vi "Actor Core.vi"(8 "error in":errorcluster, 11 "hydraharp_panel in":refnum<class "tt20panel.lvclass">) -> (0 "error out":errorcluster, 3 "Actor out":refnum<class "Actor.lvclass">)   [LabVIEW 2015, in "tt20panel.lvclass"]
doc: "(<B>Filename</B>: Actor Framework.lvlib:Actor.lvclass:Actor Core.vi)\n\nReceives messages to the actor, reacts to them, and initiates any error handling that may shut the actor down.\n\nDescendant classes may override this VI to append parallel tasks for the actor to complete while it handles messages. Overrides use the Call Parent Method node."
uses:
  tt20panel.lvclass
  <vilib>/ActorFramework/Actor/Actor.lvclass
  tt20_tasks_tdef.ctl
  tt20_settings_tdef.ctl
  tt20_ch_settings_tdef.ctl
  tt20_acq_mode_tdef.ctl
  UI/panel_class/panel.lvclass/panel.ctl
  <vilib>/ActorFramework/Actor/Actor.lvclass/Actor.ctl
  <vilib>/ActorFramework/Message Enqueuer/Message Enqueuer.lvclass/Message Enqueuer.ctl
  tt20panel.lvclass/tt20panel.ctl
  tt20_class/tt20_hardware_info_tdef.ctl
  tt20panel Messages/tt20panel_connect Msg/tt20panel_connect Msg.lvclass/tt20panel_connect Msg.ctl
  tt20panel Messages/tt20panel_DO_apply_settings Msg/tt20panel_DO_apply_settings Msg.lvclass/tt20panel_DO_apply_settings Msg.ctl
  tt20panel Messages/tt20panel_DO_chart_counts Msg/tt20panel_DO_chart_counts Msg.lvclass/tt20panel_DO_chart_counts Msg.ctl
  tt20_class/tt20_histo_settings_tdef.ctl
  tt20panel Messages/tt20panel_lifetime Msg/tt20panel_lifetime Msg.lvclass/tt20panel_lifetime Msg.ctl
  tt20panel Messages/tt20panel_correlate Msg/tt20panel_correlate Msg.lvclass/tt20panel_correlate Msg.ctl
  tt20_stream_settings_tdef.ctl
  tt20panel Messages/tt20panel_DO_stream_data Msg/tt20panel_DO_stream_data Msg.lvclass/tt20panel_DO_stream_data Msg.ctl
  <vilib>/ActorFramework/Message Enqueuer/Init from Existing Queue.vi
  <vilib>/ActorFramework/Message Enqueuer/Enqueue.vi
  <vilib>/ActorFramework/Message Priority Queue/Priority Enqueue.vi
  <vilib>/ActorFramework/Message Enqueuer/Message Enqueuer.lvclass
  tt20panel Messages/tt20panel_DO_disconnect Msg/tt20panel_DO_disconnect Msg.lvclass
  tt20panel Messages/tt20panel_connect Msg/tt20panel_connect Msg.lvclass
  tt20panel Messages/tt20panel_DO_apply_settings Msg/tt20panel_DO_apply_settings Msg.lvclass
  tt20panel Messages/tt20panel_DO_chart_counts Msg/tt20panel_DO_chart_counts Msg.lvclass
  tt20panel Messages/tt20panel_lifetime Msg/tt20panel_lifetime Msg.lvclass
  tt20panel Messages/tt20panel_correlate Msg/tt20panel_correlate Msg.lvclass
  tt20panel Messages/tt20panel_DO_stream_data Msg/tt20panel_DO_stream_data Msg.lvclass
  UI/panel_class/panel.lvclass
panel:
  in  "save_settings":bool
  in  "connect":bool
  out "Status":string
  out "error out 2":errorcluster
  in  "stop_task":bool
  in  "do_task":bool
  in  "Task":T1
  in  "tt20_tab":enum32{"Basic Settings", "File Stream"}(tab)
  in  "Number of Bins":i64
  in  "Bin Width (ps)":i64
  in  "Mode":T2
  out "Ch5":dbl
  out "Ch6":dbl
  out "Ch7":dbl
  in  "tt20_settings":T3=[{"enable"=TRUE, "trigger_level"=0.0, "deadtime_ns"=6, "delay_ps"=0}, {"enable"=TRUE, "trigger_level"=1.5, "deadtime_ns"=6, "delay_ps"=0}, {"enable"=TRUE, "trigger_level"=1.5, "deadtime_ns"=6, "delay_ps"=0}, {"enable"=FALSE, "trigger_level"=1.5, "deadtime_ns"=6, "delay_ps"=0}, {"enable"=FALSE, "trigger_level"=1.5, "deadtime_ns"=6, "delay_ps"=0}, {"enable"=FALSE, "trigger_level"=1.5, "deadtime_ns"=6, "delay_ps"=0}, {"enable"=FALSE, "trigger_level"=1.5, "deadtime_ns"=6, "delay_ps"=0}, {"enable"=FALSE, "trigger_level"=1.5, "deadtime_ns"=6, "delay_ps"=0}] {"trigger_level" min=0.0 max=5.0}
  out "Ch0":dbl
  out "Ch1":dbl
  out "Ch2":dbl
  out "Ch3":dbl
  out "Ch4":dbl
  in  "Reference Channel":u8 max=7 step=1
  in  "Stream Path":path
  in  "acq_time (s)":u32=1000
  in  "Stream Notes":string
  # "Time Tagger 20"
  # "Counts/s"
  # "Enable"
  # "Trig Lvl (V)"
  # "Dedtime (ns)"
  # "Delay (ps)"
  # "Stream Settings"
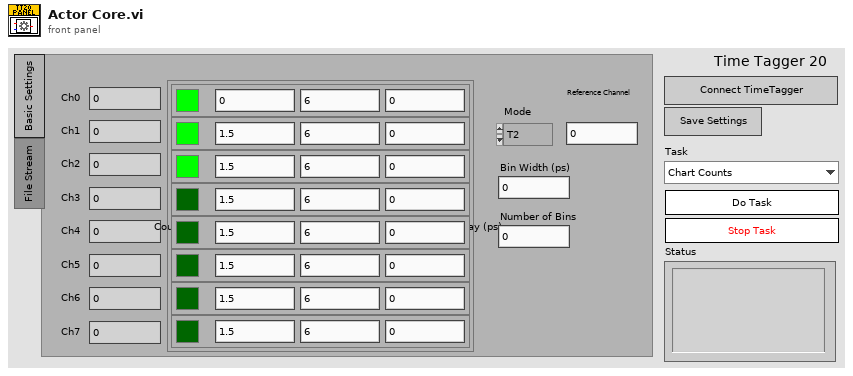
[diagram p1: front panel]
types:
  T1 = typedef "tt20_tasks_tdef.ctl" = enum16{"Chart Counts", "Stream to File", "Lifetime", "Correlate"}
  T2 = typedef "tt20_acq_mode_tdef.ctl" = enum16{"T2", "T3"}
  T3 = typedef "tt20_settings_tdef.ctl" = T4[]
  T4 = typedef "tt20_ch_settings_tdef.ctl" = cluster{"enable":bool, "trigger_level":dbl, "deadtime_ns":i64, "delay_ps":i64}
  T5 = typedef "tt20_evebnt_refs_tdef.ctl" = cluster{"info":refnum<event-registration>, "stream_done":refnum<event-registration>, "update_status":refnum<event-registration>, "update_counts":refnum<event-registration>}
  T6 = cluster{"stop_ui_ref":refnum<event-registration>, "info":refnum<event-registration>, "stream_done":refnum<event-registration>, "update_status":refnum<event-registration>, "update_counts":refnum<event-registration>}
  T7 = typedef "tt20_hardware_info_tdef.ctl" = cluster{"model":string, "serial":string, "trigger_level":dbl[], "input_delay":i64[], "deadtime":i64[], "num_channels":u32, "status":string, "enabled":bool[], "Mode":T2, "Reference Channel":u8}
  T8 = enum16{"open", "replace", "create", "open or create", "replace or create", "replace or create with confirmation"}
  T9 = enum8{"Enabled", "Disabled", "Disabled and Grayed Out"}
  T10 = typedef "tt20_histo_settings_tdef.ctl" = cluster{"click_channel":u32, "start_channel":u32, "binwidth":i64, "n_bins":i32}
  T11 = typedef "tt20_stream_settings_tdef.ctl" = cluster{"Stream Path":path, "acq_time (s)":u32, "Stream Notes":string}
  T12 = typedef "tt20_event_tdef.ctl" = cluster{"tt20_get_info":refnum<user-event>, "stream_done":refnum<user-event>, "update_status":refnum<user-event>, "update_counts":refnum<user-event>}
  T13 = cluster{"getTriggerLevel":dbl, "getInputDelay":i64, "getDeadtime":i64}
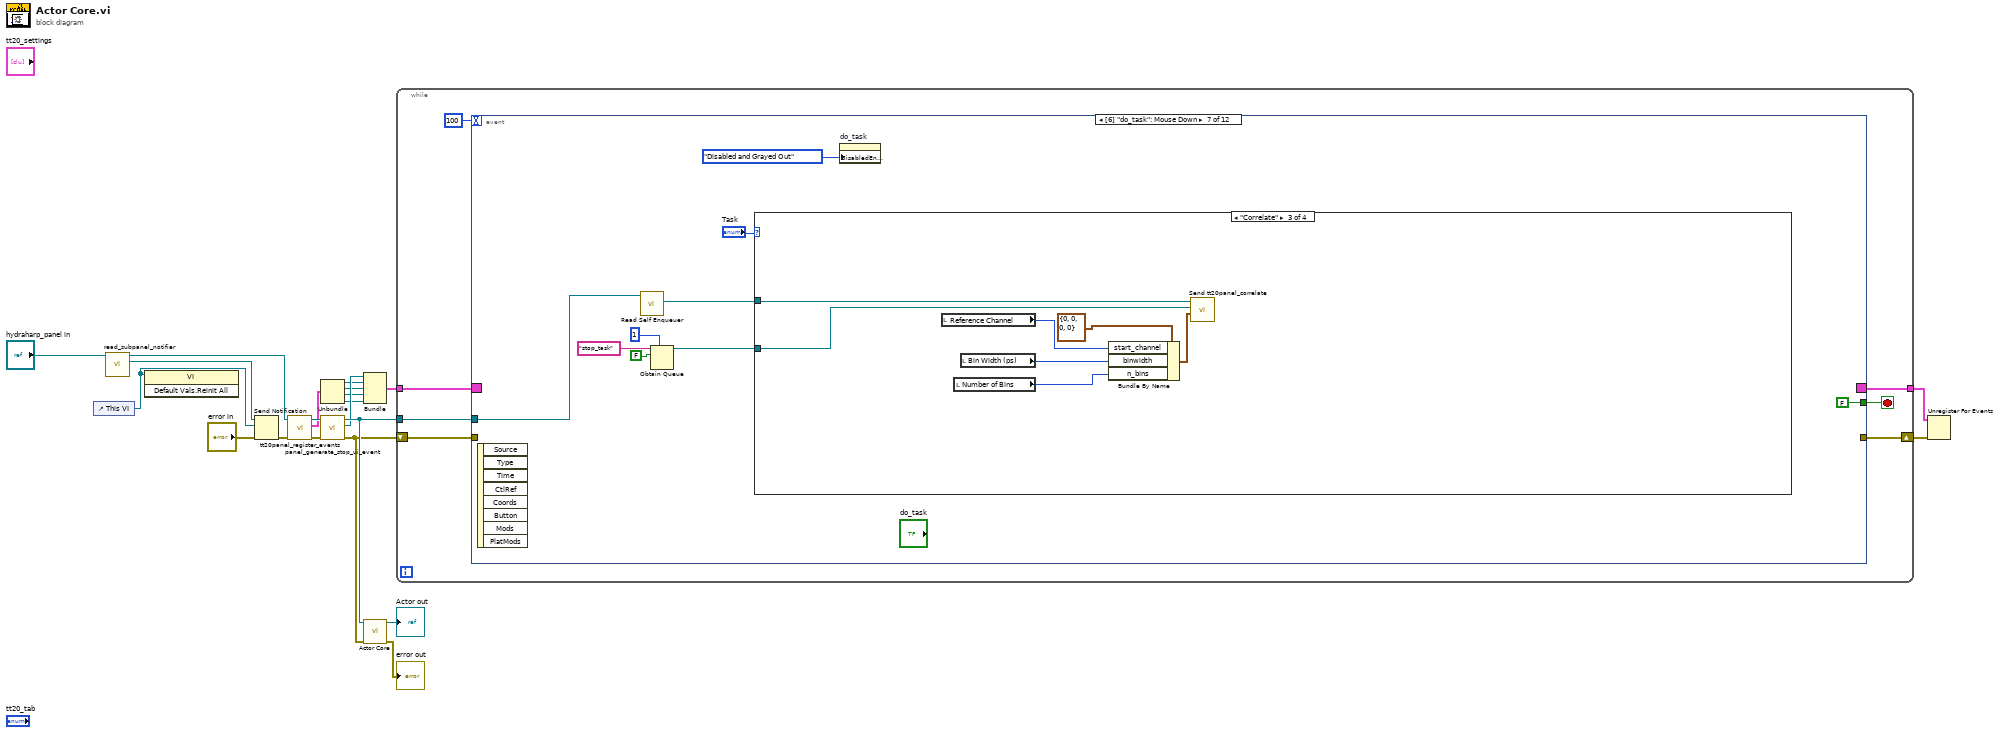
[diagram p0: block diagram]
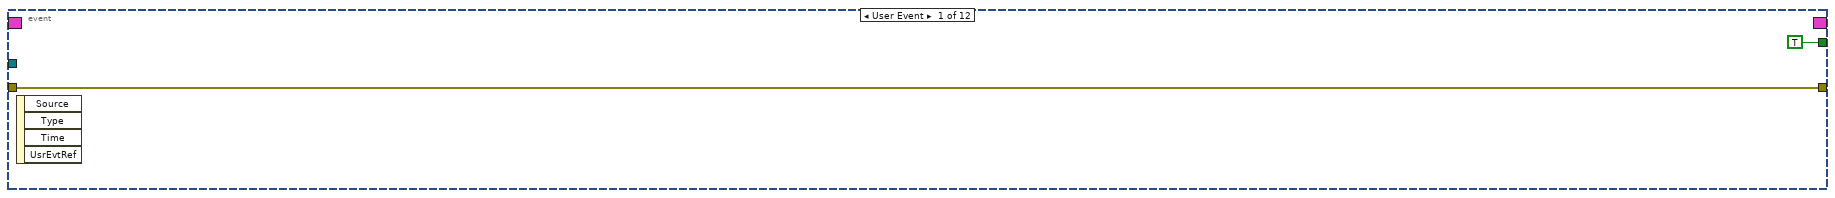
[diagram p2: hidden frame]
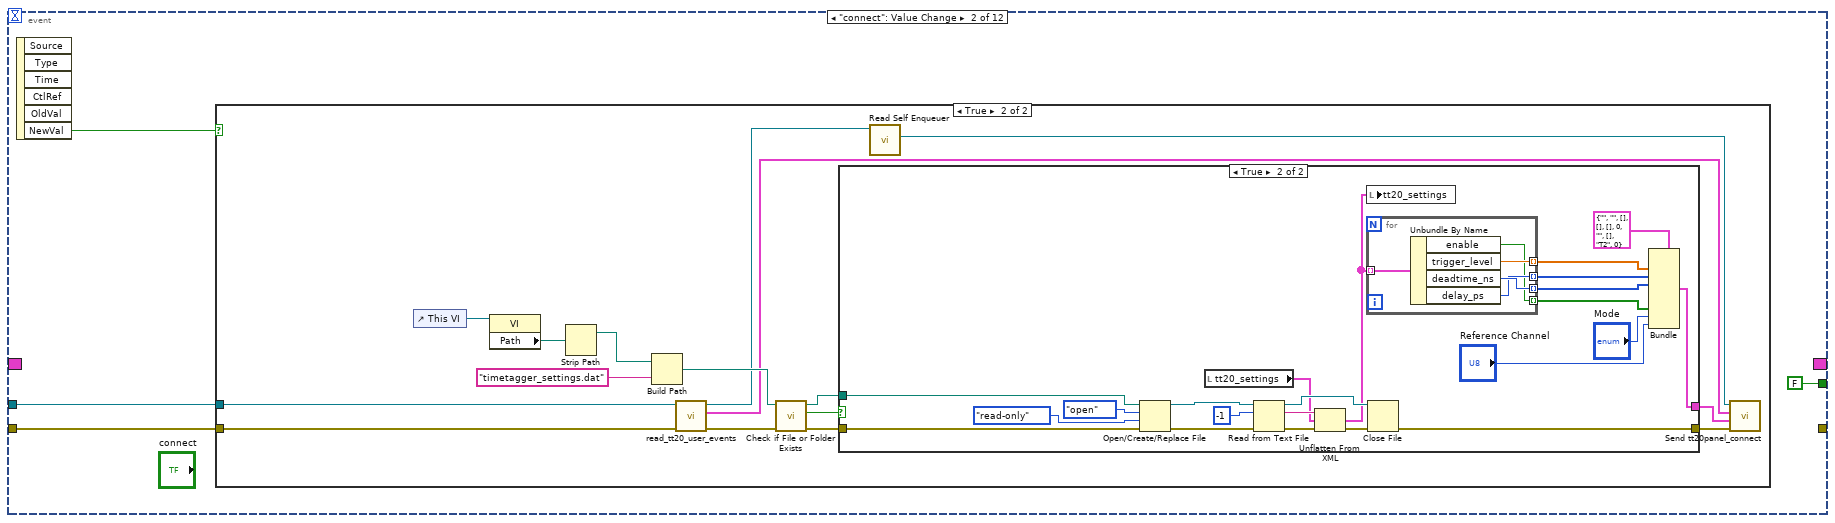
[diagram p3: hidden frame]
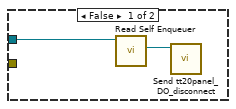
[diagram p4: hidden frame]
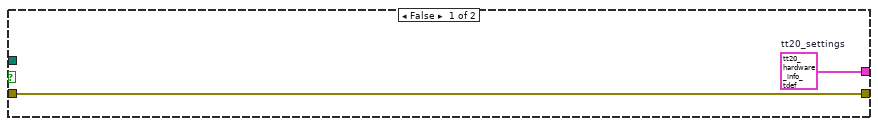
[diagram p5: hidden frame]
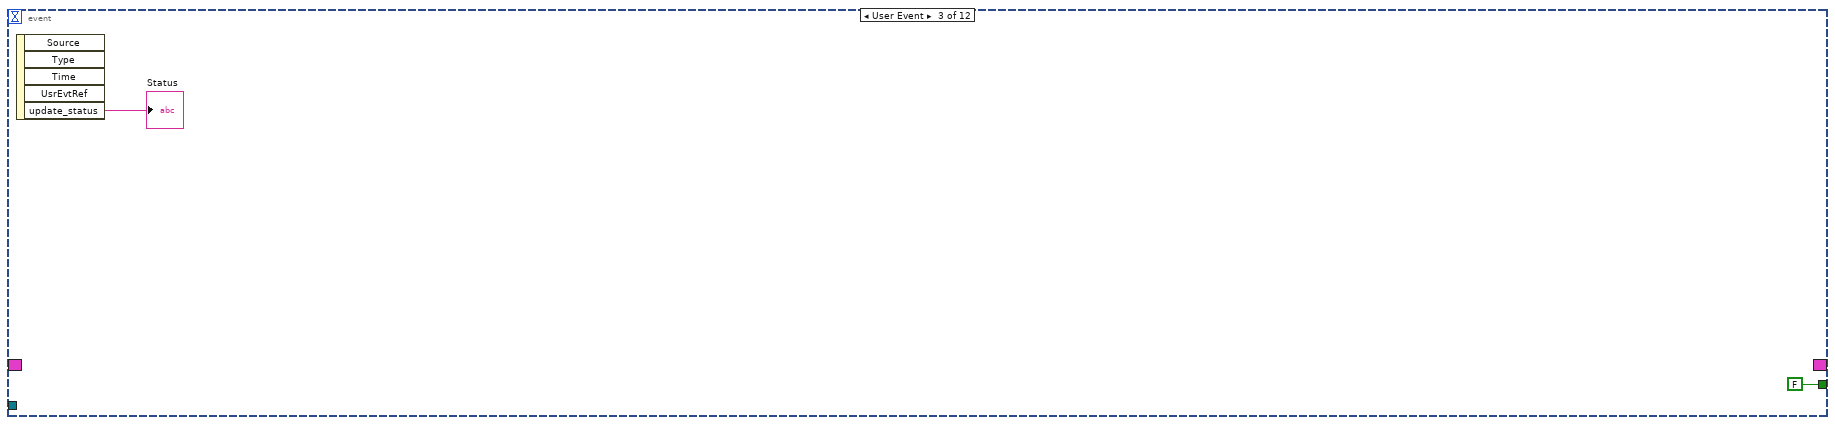
[diagram p6: hidden frame]
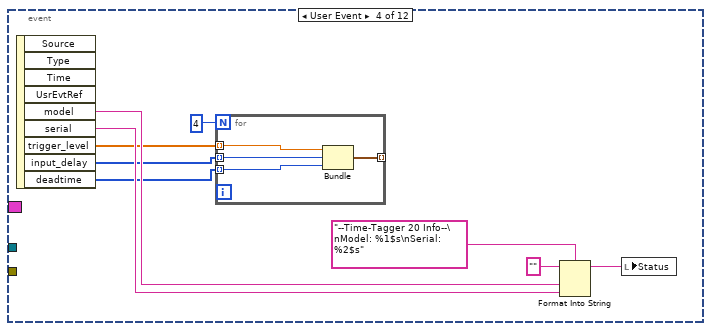
[diagram p7: hidden frame]
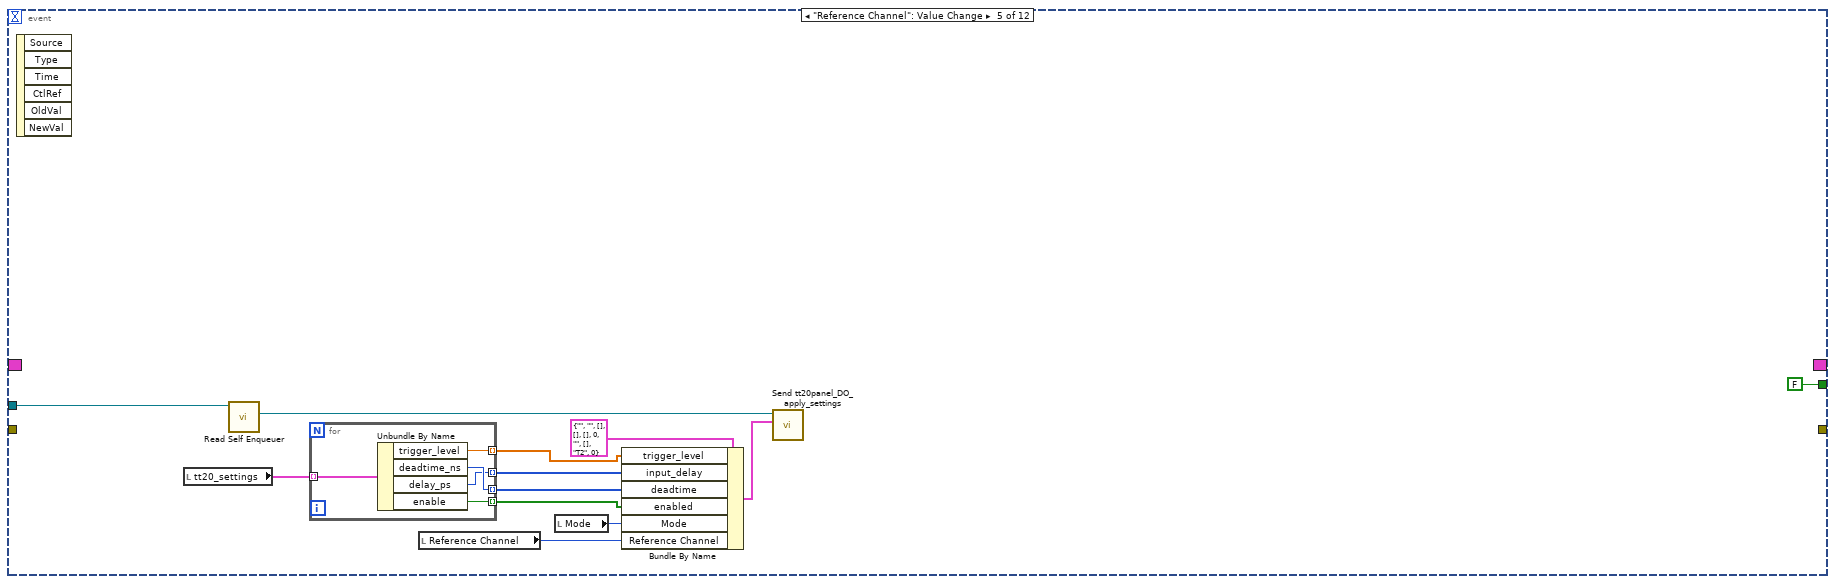
[diagram p8: hidden frame]
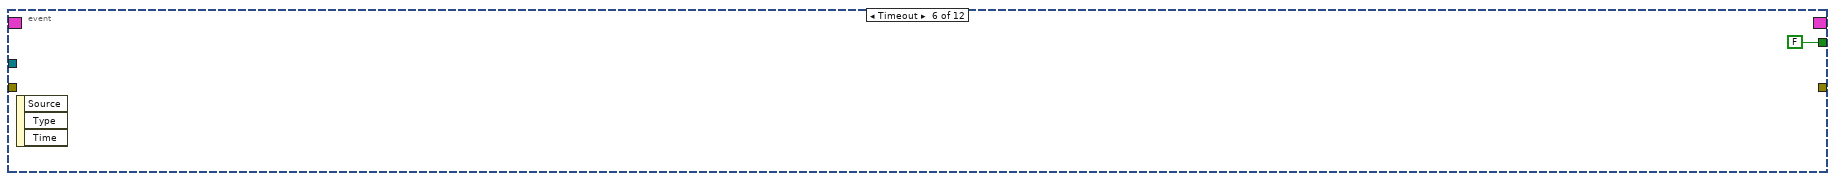
[diagram p9: hidden frame]
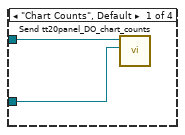
[diagram p10: hidden frame]
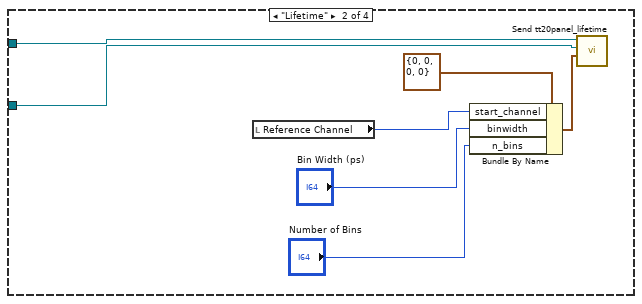
[diagram p11: hidden frame]
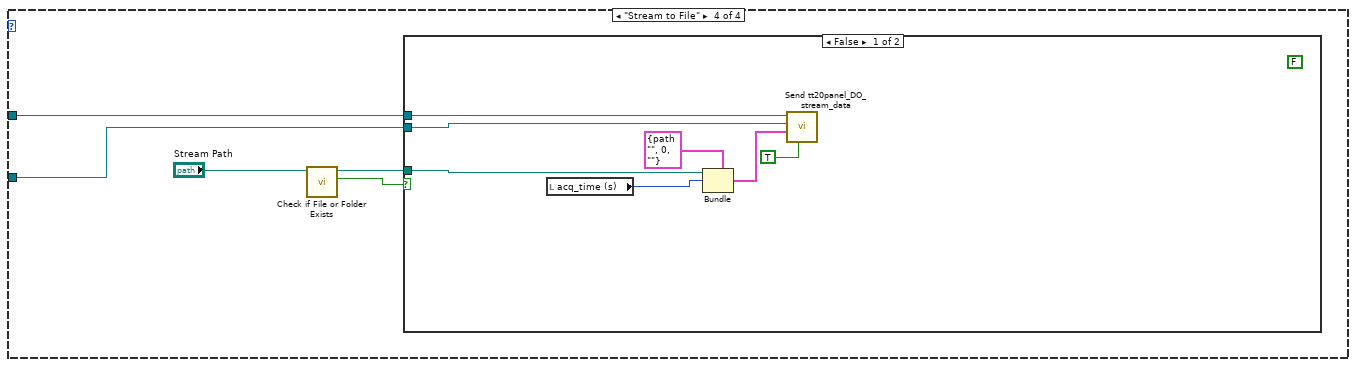
[diagram p12: hidden frame]
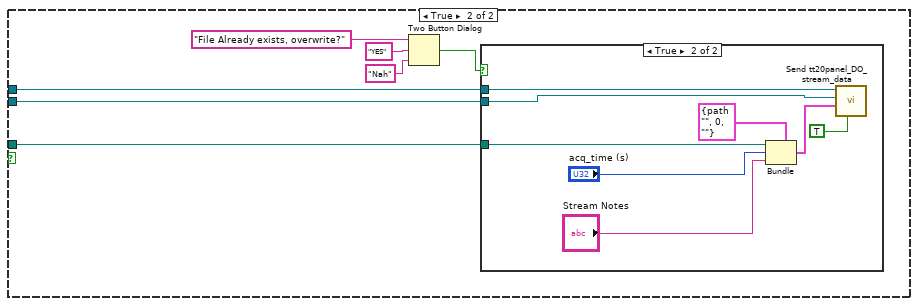
[diagram p13: hidden frame]
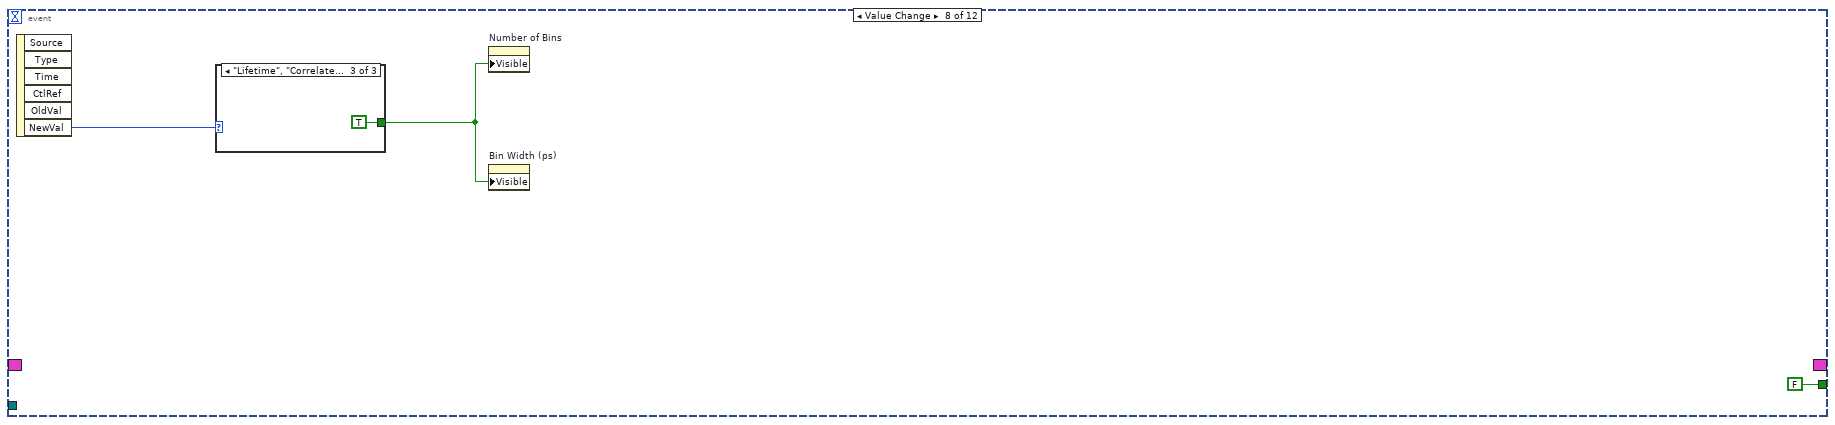
[diagram p15: hidden frame]
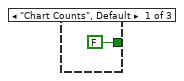
[diagram p16: hidden frame]
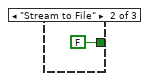
[diagram p17: hidden frame]
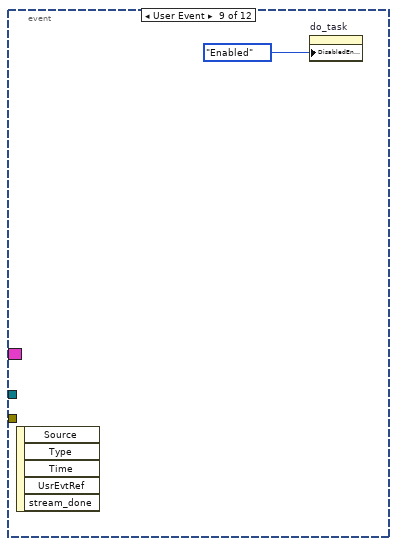
[diagram p18: hidden frame]
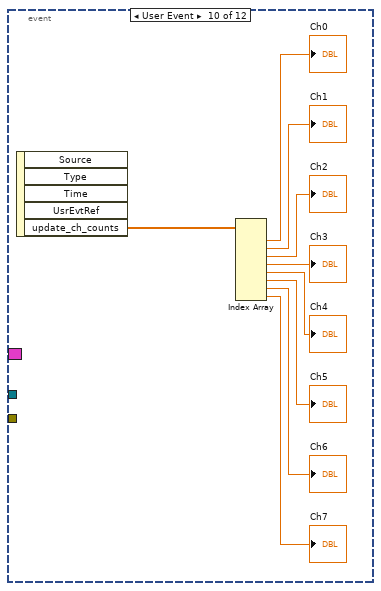
[diagram p19: hidden frame]
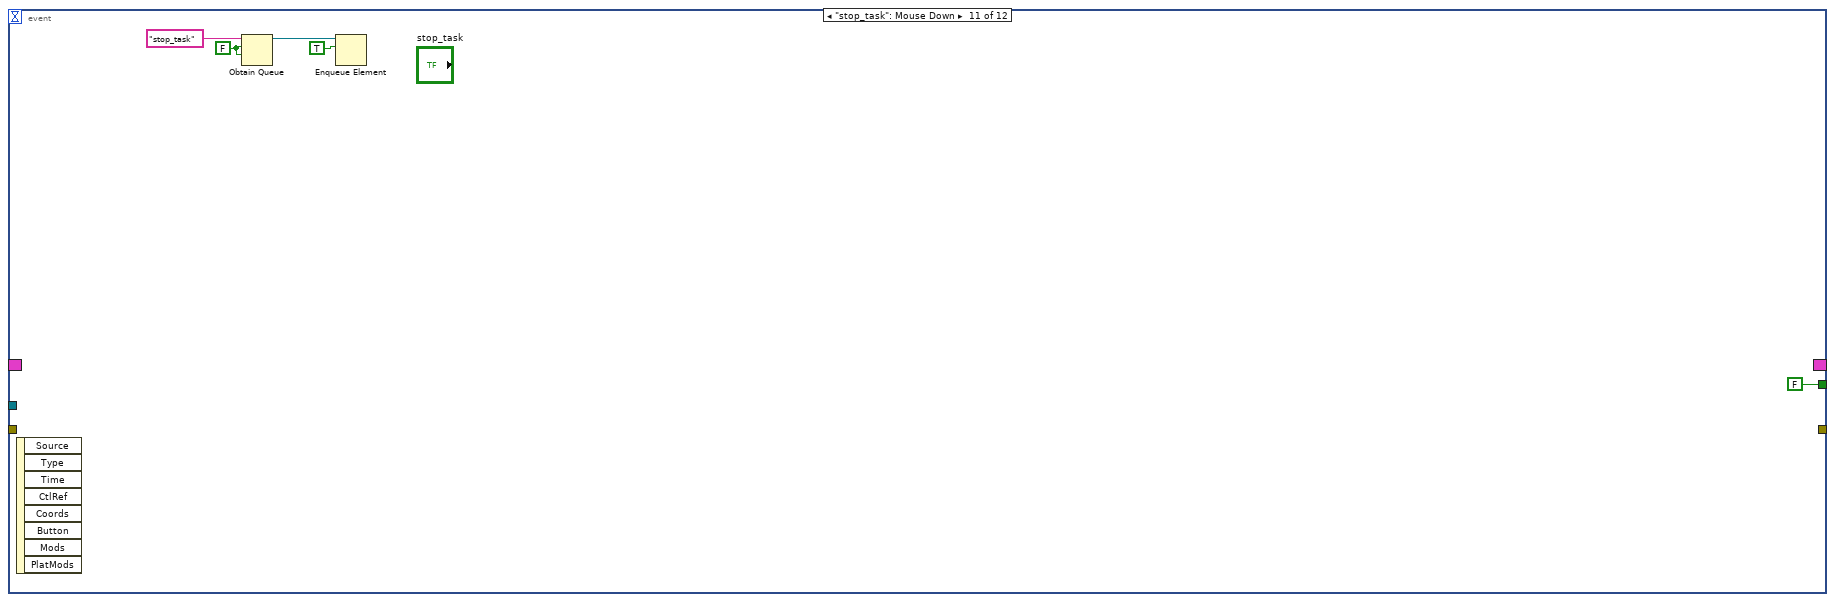
[diagram p20: hidden frame]
diagram:
  n1 = control-ref of="This VI"() -> (w16:refnum<vi>)
  n2 = call "read_subpanel_notifier.vi"("panel in"="hydraharp_panel in") -> ("subpanel_notifier"=w14:refnum<notifier>, "panel out"=w10:refnum<class "tt20panel.lvclass">)  [unwired: 8 in, 1 out]
  n3 = invoke class="VI" method="Default Vals.Reinit All"(reference=w16) -> ()  [unwired: 2 in, 3 out]
  n4 = Send Notification(notification=w16, notifier=w14, error in (no error)="error in") -> (error out=w11:errorcluster)  [unwired: 1 out]
  n5 = call "tt20panel_register_events.vi"("error in (no error)"=w11, "tt20panel in"=w10) -> ("error out"=w8:errorcluster, "event_refs"=w5:T5, "tt20panel out"=w9:refnum<class "tt20panel.lvclass">)  [unwired: 7 in]
  n6 = Unbundle(w5) -> ("info"=w4:refnum<event-registration>, "stream_done"=w3:refnum<event-registration>, "update_status"=w2:refnum<event-registration>, "update_counts"=w1:refnum<event-registration>)
  n7 = call "panel_generate_stop_ui_event.vi"("error in (no error)"=w8, "panel in"=w9) -> ("error out"=w12:errorcluster, "stop_ui_ref"=w7:refnum<event-registration>, "panel out"=w13:refnum<class "tt20panel.lvclass">)  [unwired: 7 in]
  n8 = Bundle("stop_ui_ref"=w7, "info"=w4, "stream_done"=w3, "update_status"=w2, "update_counts"=w1) -> (w6:T6)  [unwired: 1 in]
  n9 = call-parent "Actor Core.vi"("error in"=w12, "Actor in"=w13) -> ("error out"=→"error out":errorcluster, "Actor out"=→"Actor out":refnum<class "Actor.lvclass">)  [unwired: 8 in]
  n10 = while {
    tunnel: [w28] -> w18
    shift-right: [w25] -> w17
    shift-left: w12 -> [w26]
    tunnel: w13 -> [w24]
    tunnel: w6 -> [w22]
    stop <- w27 stop-if-true
    n11 = event shown="[6] \"do_task\": Mouse Down" {
      selector: w22 -> [_ _ _ _ _ _ _ _ _ _ _ _]
      dyn-events: [_ _ _ _ _ _ _ _ _ _ _ _] -> w28
      timeout: 100 -> [_ _ _ _ _ _ _ _ _ _ _ _]
      tunnel: [TRUE FALSE FALSE _ FALSE FALSE FALSE FALSE _ _ FALSE FALSE] -> w27
      tunnel: w26 -> [w29 w33 _ _ _ _ _ _ _ _ _ _]
      tunnel: [w29 _ _ _ _ _ _ _ _ _ _ _] -> w25
      tunnel: w24 -> [_ w34 _ _ w108 _ w122 _ _ _ _ _]
      event User Event {
        n12 = event-data() -> ()  [unwired: 1 in, 4 out]
      }
      event "connect": Value Change {
        n13 = event-data() -> ("NewVal"=w32:bool)  [unwired: 1 in, 5 out]
        n14 = case shown="True" w32 {
          tunnel: w34 -> [w36 w52]
          tunnel: w33 -> [_ w51]
          frame False {
            n15 = call <vilib>:"Read Self Enqueuer.vi"("Actor"=w36) -> ("Self Enqueuer"=w35:refnum<class "Message Enqueuer.lvclass">)  [unwired: 10 in]
            n16 = call "Send tt20panel_DO_disconnect.vi"("Message Enqueuer"=w35) -> ()  [unwired: 9 in, 2 out]
          }
          frame True {
            n17 = control-ref of="This VI"() -> (w50:refnum<vi>)
            n18 = property class="VI"(reference=w50) -> ("Path"=w49:path)  [unwired: 1 in, 2 out]
            n19 = Strip Path(path=w49) -> (stripped path=w48:path)  [unwired: 1 out]
            n20 = Build Path(base path=w48, name or relative path="timetagger_settings.dat") -> (appended path=w46:path)
            n21 = call "read_tt20_user_events.vi"("error in (no error)"=w51, "tt20panel in"=w52) -> ("error out"=w42:errorcluster, "tt20_events"=w40:T12, "tt20panel out"=w39:refnum<class "tt20panel.lvclass">)  [unwired: 7 in]
            n22 = call <vilib>:"Check if File or Folder Exists.vi"("error in (no error)"=w42, "path"=w46) -> ("error out"=w43:errorcluster, "file or folder exists?"=w45:bool, "dup path"=w44:path)  [unwired: 7 in]
            n23 = case shown="True" w45 {
              tunnel: w44 -> [_ w76]
              tunnel: w43 -> [w53 w75]
              tunnel: [w54 w74] -> w41
              tunnel: [w53 w73] -> w37
              frame False {
                w54 = T7 {"model"="", "serial"="", "trigger_level"=[0.15, 0.15, 0.15, 0.15, 0.15], "input_delay"=[6, 6, 6, 6, 6], "deadtime"=[0, 0, 0, 0, 0], "num_channels"=0, "status"="", "enabled"=[], "Mode"=enum."T2", "Reference Channel"=0}  # tt20_settings
              }
              frame True {
                n24 = Open/Create/Replace File(file path (use dialog)=w76, error in=w75, operation (0:open)=T8."open", access (0:read/write)=enum16{"read/write", "read-only", "write-only"}."read-only") -> (refnum out=w66:refnum<file>, error out=w65:errorcluster)  [unwired: 2 in, 1 out]
                n25 = local read "tt20_settings"() -> (w58:T3)
                n26 = Read from Text File(file (use dialog)=w66, count=-1, error in=w65) -> (refnum out=w63:refnum<file>, text=w59:string, error out=w61:errorcluster)  [unwired: 1 in, 1 out]
                n27 = Unflatten From XML(xml string=w59, type=w58, error in (no error)=w61) -> (value=w55:T3, error out=w60:errorcluster)
                n28 = local write "tt20_settings"(w55) -> ()
                n29 = for {
                  tunnel: w55 -> [w81] mode=indexing
                  tunnel: [w80] -> w70 mode=indexing
                  tunnel: [w79] -> w69 mode=indexing
                  tunnel: [w78] -> w68 mode=indexing
                  tunnel: [w77] -> w62 mode=indexing
                  n30 = Unbundle By Name(w81) -> ("enable"=w77:bool, "trigger_level"=w80:dbl, "deadtime_ns"=w79:i64, "delay_ps"=w78:i64)
                }
                n31 = Close File(refnum=w63, error in=w60) -> (error out=w73:errorcluster)  [unwired: 1 out]
                n32 = Bundle(cluster=T7 {"model"="", "serial"="", "trigger_level"=[], "input_delay"=[], "deadtime"=[], "num_channels"=0, "status"="", "enabled"=[], "Mode"=enum."T2", "Reference Channel"=0} ("tt20_settings"), "trigger_level"=w70, "input_delay"=w68, "deadtime"=w69, "enabled"=w62, "Mode"="Mode", "Reference Channel"="Reference Channel") -> (w74:T7)  [unwired: 4 in]
              }
            }
            n33 = call <vilib>:"Read Self Enqueuer.vi"("Actor"=w39) -> ("Self Enqueuer"=w38:refnum<class "Message Enqueuer.lvclass">)  [unwired: 10 in]
            n34 = call "Send tt20panel_connect.vi"("error in (no error)"=w37, "tt20_settings"=w41, "tt20_events"=w40, "Message Enqueuer"=w38) -> ()  [unwired: 6 in, 2 out]
          }
        }
      }
      event User Event {
        n35 = event-data() -> ("update_status"=→"Status":string)  [unwired: 1 in, 4 out]
      }
      event User Event {
        n36 = event-data() -> ("model"=w92:string, "serial"=w91:string, "trigger_level"=w87:dbl[], "input_delay"=w85:i64[], "deadtime"=w86:i64[])  [unwired: 1 in, 4 out]
        n37 = for {
          N: 4 -> [_]
          tunnel: w87 -> [w96] mode=indexing
          tunnel: w86 -> [w94] mode=indexing
          tunnel: w85 -> [w95] mode=indexing
          tunnel: [w93] -> _ mode=indexing
          n38 = Bundle("getTriggerLevel"=w96, "getInputDelay"=w95, "getDeadtime"=w94) -> (w93:T13)  [unwired: 1 in]
        }
        n39 = Format Into String(format string="--Time-Tagger 20 Info--\nModel: %1$s\nSerial: %2$s", initial string="", w92, w91) -> (resulting string=w88:string)  [unwired: 1 in, 1 out]
        n40 = local write "Status"(w88) -> ()
      }
      event "Reference Channel": Value Change {
        n41 = event-data() -> ()  [unwired: 1 in, 6 out]
        n42 = local read "tt20_settings"() -> (w97:T3)
        n43 = call <vilib>:"Read Self Enqueuer.vi"("Actor"=w108) -> ("Self Enqueuer"=w106:refnum<class "Message Enqueuer.lvclass">)  [unwired: 10 in]
        n44 = for {
          tunnel: w97 -> [w113] mode=indexing
          tunnel: [w112] -> w103 mode=indexing
          tunnel: [w111] -> w101 mode=indexing
          tunnel: [w110] -> w102 mode=indexing
          tunnel: [w109] -> w100 mode=indexing
          n45 = Unbundle By Name(w113) -> ("trigger_level"=w112:dbl, "deadtime_ns"=w111:i64, "delay_ps"=w110:i64, "enable"=w109:bool)
        }
        n46 = local read "Reference Channel"() -> (w98:u8)
        n47 = local read "Mode"() -> (w99:T2)
        n48 = Bundle By Name(cluster=T7 {"model"="", "serial"="", "trigger_level"=[], "input_delay"=[], "deadtime"=[], "num_channels"=0, "status"="", "enabled"=[], "Mode"=enum."T2", "Reference Channel"=0} ("tt20_settings"), "trigger_level"=w103, "input_delay"=w102, "deadtime"=w101, "enabled"=w100, "Mode"=w99, "Reference Channel"=w98) -> (w104:T7)
        n49 = call "Send tt20panel_DO_apply_settings.vi"("tt20_settings"=w104, "Message Enqueuer"=w106) -> ()  [unwired: 8 in, 2 out]
      }
      event Timeout {
        n50 = event-data() -> ()  [unwired: 1 in, 3 out]
      }
      event "do_task": Mouse Down {
        n51 = event-data() -> ()  [unwired: 1 in, 8 out]
        n52 = call <vilib>:"Read Self Enqueuer.vi"("Actor"=w122) -> ("Self Enqueuer"=w121:refnum<class "Message Enqueuer.lvclass">)  [unwired: 10 in]
        n53 = Obtain Queue(max queue size (-1, unlimited)=1, name (unnamed)="stop_task", element data type=FALSE) -> (queue out=w116:refnum<queue>)  [unwired: 2 in, 2 out]
        n54 = case shown="\"Correlate\"" "Task" {
          tunnel: w121 -> [w125 w132 w139 w142]
          tunnel: w116 -> [w124 w131 w138 w141]
          frame "Chart Counts", Default {
            n55 = call "Send tt20panel_DO_chart_counts.vi"("stop_counts"=w124, "Message Enqueuer"=w125) -> ()  [unwired: 8 in, 2 out]
          }
          frame "Lifetime" {
            n56 = local read "Reference Channel"() -> (w129:u8)
            n57 = Bundle By Name(cluster=T10 {"click_channel"=0, "start_channel"=0, "binwidth"=0, "n_bins"=0} ("histo_settings"), "start_channel"=w129, "binwidth"="Bin Width (ps)", "n_bins"="Number of Bins") -> (w126:T10)
            n58 = call "Send tt20panel_lifetime.vi"("histo_settings"=w126, "stop_counts"=w131, "Message Enqueuer"=w132) -> ()  [unwired: 7 in, 2 out]
          }
          frame "Correlate" {
            n59 = local read "Reference Channel"() -> (w133:u8)
            n60 = local read "Number of Bins"() -> (w135:i64)
            n61 = local read "Bin Width (ps)"() -> (w136:i64)
            n62 = Bundle By Name(cluster=T10 {"click_channel"=0, "start_channel"=0, "binwidth"=0, "n_bins"=0} ("histo_settings"), "start_channel"=w133, "binwidth"=w136, "n_bins"=w135) -> (w134:T10)
            n63 = call "Send tt20panel_correlate.vi"("histo_settings"=w134, "stop_counts"=w138, "Message Enqueuer"=w139) -> ()  [unwired: 7 in, 2 out]
          }
          frame "Stream to File" {
            n64 = call <vilib>:"Check if File or Folder Exists.vi"("path"="Stream Path") -> ("file or folder exists?"=w143:bool, "dup path"=w140:path)  [unwired: 8 in, 1 out]
            n65 = case shown="False" w143 {
              tunnel: w142 -> [w147 w154]
              tunnel: w141 -> [w146 w153]
              tunnel: w140 -> [w148 w152]
              frame False {
                (unwired) FALSE ("T button?")
                n66 = local read "acq_time (s)"() -> (w149:u32)
                n67 = Bundle(cluster=T11 {"Stream Path"=path "", "acq_time (s)"=0, "Stream Notes"=""} ("output cluster"), "Stream Path"=w148, "acq_time (s)"=w149) -> (w150:T11)  [unwired: 1 in]
                n68 = call "Send tt20panel_DO_stream_data.vi"("Overwrite?"=TRUE, "stream_settings"=w150, "stop_counts"=w146, "Message Enqueuer"=w147) -> ()  [unwired: 6 in, 2 out]
              }
              frame True {
                n69 = Two Button Dialog(message="File Already exists, overwrite?", 1:"Nah" ("F button name (\"Cancel\")"), 2:"YES" ("T button name (\"OK\")")) -> (T button?=w155:bool)
                n70 = case shown="True" w155 {
                  tunnel: w154 -> [_ w162]
                  tunnel: w153 -> [_ w161]
                  tunnel: w152 -> [_ w159]
                  frame False {
                  }
                  frame True {
                    n71 = Bundle(cluster=T11 {"Stream Path"=path "", "acq_time (s)"=0, "Stream Notes"=""} ("output cluster"), "Stream Path"=w159, "acq_time (s)"="acq_time (s)", "Stream Notes"="Stream Notes") -> (w163:T11)
                    n72 = call "Send tt20panel_DO_stream_data.vi"("Overwrite?"=TRUE, "stream_settings"=w163, "stop_counts"=w161, "Message Enqueuer"=w162) -> ()  [unwired: 6 in, 2 out]
                  }
                }
              }
            }
          }
        }
        n73 = property on="do_task" class="Bool (strict)"("DisabledEnum"=T9."Disabled and Grayed Out" ("Disabled")) -> ()  [unwired: 2 in, 2 out]
      }
      event Value Change {
        n74 = event-data() -> ("NewVal"=w169:T1)  [unwired: 1 in, 5 out]
        n75 = case shown="\"Lifetime\", \"Correlate\"" w169 {
          tunnel: [FALSE ("Visible") FALSE ("Visible") TRUE ("Visible")] -> w167
          frame "Chart Counts", Default {
          }
          frame "Stream to File" {
          }
          frame "Lifetime", "Correlate" {
          }
        }
        n76 = property on="Number of Bins" class="DigNum (strict)"("Visible"=w167) -> ()  [unwired: 2 in, 2 out]
        n77 = property on="Bin Width (ps)" class="DigNum (strict)"("Visible"=w167) -> ()  [unwired: 2 in, 2 out]
      }
      event User Event {
        n78 = event-data() -> ()  [unwired: 1 in, 5 out]
        n79 = property on="do_task" class="Bool (strict)"("DisabledEnum"=T9."Enabled" ("Disabled")) -> ()  [unwired: 2 in, 2 out]
      }
      event User Event {
        n80 = event-data() -> ("update_ch_counts"=w182:dbl[])  [unwired: 1 in, 4 out]
        n81 = Index Array(array=w182) -> (element #1=→"Ch0":dbl, element #2=→"Ch1":dbl, element #3=→"Ch2":dbl, element #4=→"Ch3":dbl, element #5=→"Ch4":dbl, element #6=→"Ch5":dbl, element #7=→"Ch6":dbl, element #8=→"Ch7":dbl)  [unwired: 8 in]
      }
      event "stop_task": Mouse Down {
        w186 = FALSE ("create if not found? (T)")
        n82 = event-data() -> ()  [unwired: 1 in, 8 out]
        n83 = Obtain Queue(name (unnamed)="stop_task", element data type=w186, create if not found? (T)=w186) -> (queue out=w185:refnum<queue>)  [unwired: 2 in, 2 out]
        n84 = Enqueue Element(queue=w185, element=TRUE) -> ()  [unwired: 2 in, 3 out]
      }
      event "save_settings": Mouse Down {
        n85 = event-data() -> ()  [unwired: 1 in, 8 out]
        n86 = control-ref of="This VI"() -> (w203:refnum<vi>)
        n87 = property class="VI"(reference=w203) -> ("Path"=w202:path)  [unwired: 1 in, 2 out]
        n88 = Strip Path(path=w202) -> (stripped path=w201:path)  [unwired: 1 out]
        n89 = local read "tt20_settings"() -> (w194:T3)
        n90 = Build Path(base path=w201, name or relative path="timetagger_settings.dat") -> (appended path=w200:path)
        n91 = Flatten To XML(anything=w194) -> (xml string=w193:string)
        n92 = Open/Create/Replace File(file path (use dialog)=w200, operation (0:open)=T8."replace or create") -> (refnum out=w195:refnum<file>, error out=w192:errorcluster)  [unwired: 4 in, 1 out]
        n93 = Write to Text File(file (use dialog)=w195, text=w193, error in=w192) -> (refnum out=w189:refnum<file>, error out=w191:errorcluster)  [unwired: 1 in, 1 out]
        n94 = Flush File(refnum=w189, error in=w191) -> (refnum out=w188:refnum<file>, error out=w190:errorcluster)
        n95 = Close File(refnum=w188, error in=w190) -> (error out=→"error out 2":errorcluster)  [unwired: 1 out]
      }
    }
  }
  n96 = Unregister For Events(event registration refnum=w18, error in=w17) -> ()  [unwired: 1 out]
